vi "IR_Team_V_1.vi"() -> ()   [LabVIEW 2014]
doc: "The myRIO v1.1 FPGA Shipping Personality. This personality contains support for:\n- 2 Analog Input Interrupt channel\n- 4 Digital Input Interrupt channel\n- 1 Timer\n- 1 Accelerometer\n- 1 Button\n- 4 LED\n- 10 Analog Input channels with 1 Sample\n- 6 Analog Output channels with 1 Sample\n- 40 Digital I/O channels with 1 Sample\n- 2 I2C channels\n- 4 Encoder channels\n- 6 PWM channels\n- 2 SPI channels"
uses:
  <vilib>/rvi/Emulation/niFpgaGetClockAttributes.vi
  <vilib>/rvi/Emulation/niFpgaSctlEmulationGetInTimedLoop.vi
  <vilib>/rvi/Emulation/niFpgaEmulationReportErrorSimple.vi
  <vilib>/rvi/Emulation/niFpgaProcessEmulError.vi
  <vilib>/rvi/Emulation/niFpgaCriticalErrorInLSC.vi
  <vilib>/rvi/eio/common/nirviEmuTemplateMethod_errors.vi
  <vilib>/rvi/Emulation/niFpgaEmulationIsFPGAContextNoSignature.vi
  <vilib>/rvi/errors/niFpgaSetErrorForExecOnDevCompSimple.vi
  <vilib>/rvi/eio/common/nirviEmuReportErrorAndStop.vi
  <vilib>/rvi/DataTransferAndStorage/Container/Common/niFpgaContainerGetUniqueNameForEmu.vi
  <vilib>/rvi/FIFO/Fifo_Resource/nirvififoEmulationSetSize.vi
  <vilib>/rvi/FIFO/Fifo_Resource/nirviFifoEmulationQueueMgr.vi
  <instcachedir>/0/nirviFifoEmulationQueueMgr_E5CAEC123FF24DC58D834DCA3CDAA9B5.lvgen/nirviFifoEmulationQueueMgr_E5CAEC123FF24DC58D834DCA3CDAA9B5_002.vi
  <vilib>/rvi/FIFO/Fifo_Resource/nirvififoEmulationDetermineInputValidOut.vi
  <vilib>/rvi/FIFO/Fifo_Resource/nirvififoEmulationCreateLock.vi
  <vilib>/rvi/FIFO/Fifo_Resource/nirvififoEmulationObtainLock.vi
  <vilib>/rvi/FIFO/Fifo_Resource/nirvififoEmulationReleaseLock.vi
  <vilib>/rvi/occurrence/nirviWaitOnOccurrenceBase.vi
  <vilib>/rvi/errors/nirviReportUnexpectedCaseInternalError.vi
  <vilib>/rvi/errors/nirviReportUnexpectedCaseInternalError (U32).vi
  <vilib>/rvi/DataTransferAndStorage/Container/Common/niFpgaContainerSetEmuInfo.vi
  <vilib>/rvi/DataTransferAndStorage/Container/Common/niFpgaContainerExecOnDevCompGetState.vi
  <vilib>/Utility/error.llb/Clear Errors.vi
  <vilib>/rvi/interface/RandomDataEmulation/niFpgaRandomDataHandleErrors.vi
  <vilib>/eio/EIONode/EIONode.xnode
  <vilib>/rvi/DataTransferAndStorage/Container/XNode/niFpgaContainer.xnode
  <vilib>/rvi/FIFO/Fifo_Resource/nirvififoEmulationWrite.vi
  <vilib>/rvi/LocalResourceManager/LocalResourceManager.xnode
  <vilib>/rvi/FIFO/Fifo_Resource/niFpgaFifoEmulationRefIn.vi
panel:
  in  "?":enum32{"PLOT", "VALUES"}(tab)
  out "?":u16(graph)
  out "Indicator":u8(knob) scale=0.0..200.0
  out "Direct Output":u16
  out "Converted Output":u8
  out "Boolean":bool
  in  "?":bool
  out "SYS.AI.RDY":bool
  out "SYS.ACC.RDY":bool
  out "SYS.RDY":bool
  # "IR TEAM"
  # "Graph"
  # "Value"
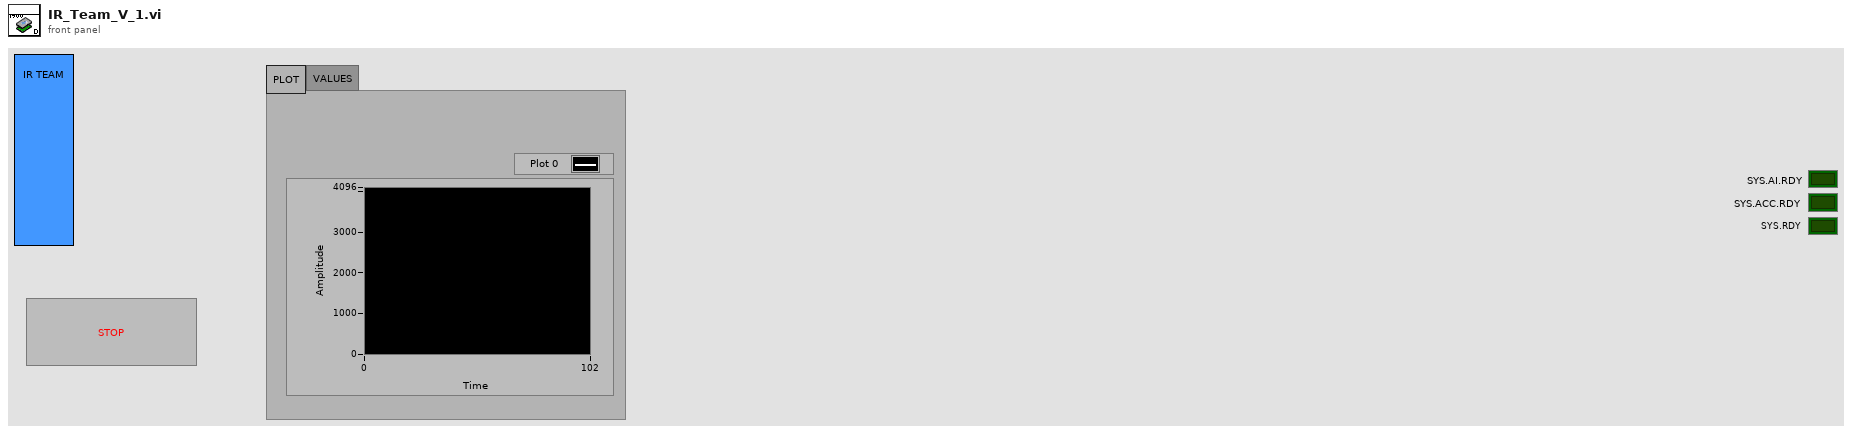
[diagram p1: front panel]
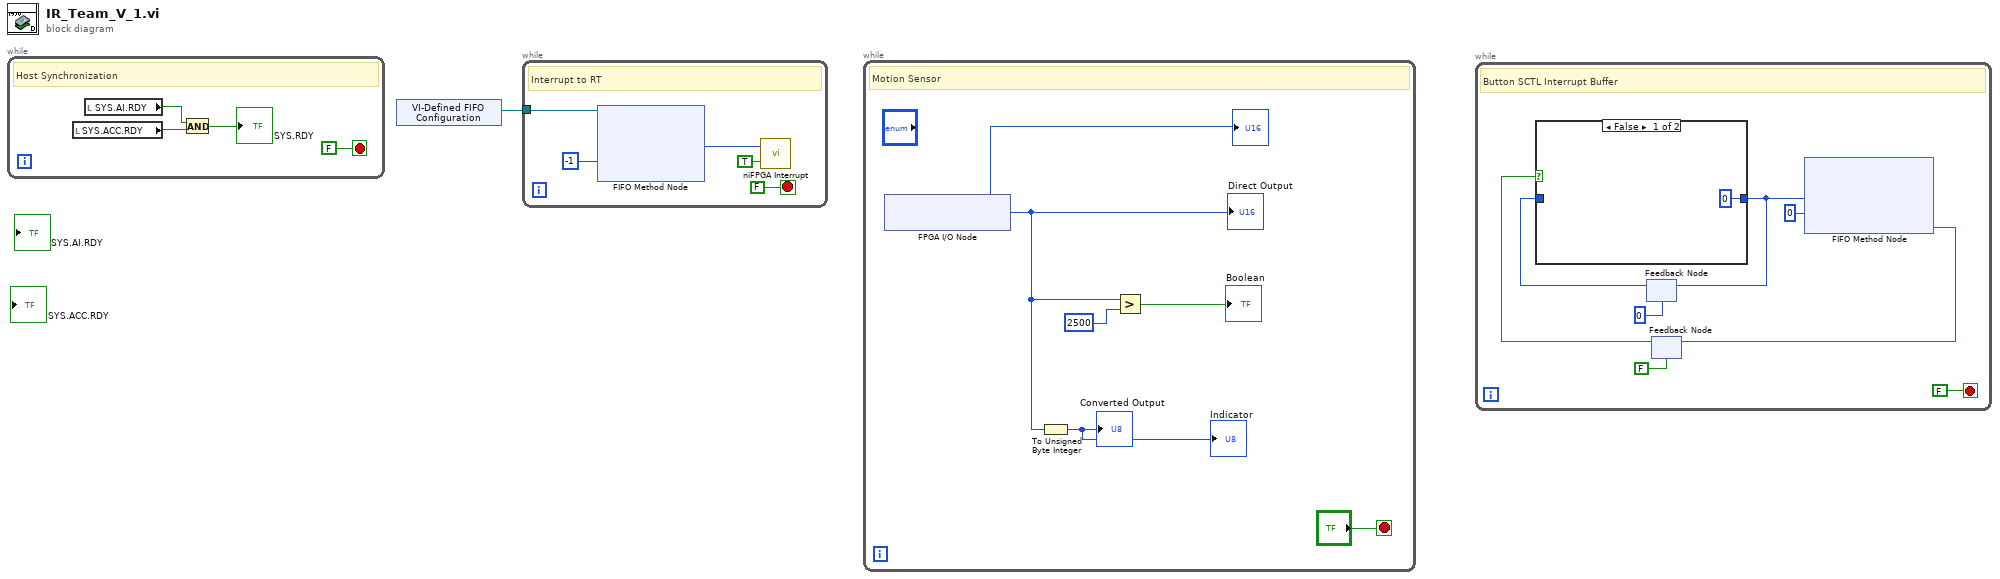
[diagram p0: block diagram]
diagram:
  n1 = while {
    stop <- FALSE stop-if-true
    # "Host Synchronization"
    n2 = local read "SYS.ACC.RDY"() -> (w3:bool)
    n3 = local read "SYS.AI.RDY"() -> (w5:bool)
    n4 = Compound Arithmetic op=AND(w5, w3) -> (→"SYS.RDY":bool)
  }
  n5 = xnode "VI-Defined FIFO Configuration"() -> ("FIFO Out"=w1:refnum<k21>)
  n6 = while {
    tunnel: w1 -> [w6]
    stop <- FALSE stop-if-true
    # "Interrupt to RT"
    n7 = xnode ("FIFO Method Node")("Timeout"=-1, "FIFO In"=w6) -> ("Element"=w9:u8)  [unwired: 2 out]
    n8 = call <vilib>:"niFPGA Interrupt.vi"("Wait Until Cleared (F)"=TRUE, "IRQ Number (0)"=w9) -> ()  [unwired: 1 in]
  }
  n9 = while "While-Schleife" {
    stop <- "?" stop-if-true
    # "Motion Sensor"
    n10 = xnode "FPGA I/O Node"() -> ("ConnectorA/AI0"=w15:u16)  [unwired: 1 in, 1 out]
    "?" <- w15
    "Direct Output" <- w15
    n11 = To Unsigned Byte Integer(number=w15) -> (unsigned 8bit integer=→"Converted Output" →"Indicator":u8)
    n12 = Greater?(x=w15, y=u16 2500) -> (0:→"Boolean":bool)
  }
  n13 = while {
    stop <- FALSE stop-if-true
    # "Button SCTL Interrupt Buffer"
    n14 = feedback #1(u8 0 ("Element")) -> (w18:u8)
    n15 = feedback #2(FALSE ("Timed Out?")) -> (w22:bool)
    n16 = case shown="False" w22 {
      tunnel: [u8 0 ("Element") w25] -> w19
      tunnel: w18 -> [_ w25]
      frame False {
      }
      frame True {
      }
    }
    n17 = feedback-in #1(w19) -> ()
    n18 = xnode ("FIFO Method Node")("Element"=w19, "Timeout"=0) -> ("Timed Out?"=w20:bool)  [unwired: 1 in, 1 out]
    n19 = feedback-in #2(w20) -> ()
  }
